vi "EdgeRegistration and ObjectTracking.vi"(8 "error in (no error)":errorcluster, 9 "Edge and object Parameters":T1={"Canny Edge Parameters"={"Sigma"=1.0, "HThresh"=0.7, "LThres"=0.2, "WindowSize"=9}, "Smoothing parameters"={"X Size"=3, "Y Size"=3, "% Tolerance"=40}, "Dilation iteration"=1, "Object recognition parameters"={"Objects"=0, "Threshold"=128, "Reject Border"=FALSE, "Fill Holes"=FALSE, "Min Object Size"=FALSE, "Min Size"=3, "Max Object Size"=FALSE, "Max Size"=100, "Show Search Area"=FALSE, "Show Center"=TRUE, "Show Bounding Box"=TRUE}} {"Object recognition parameters"."Objects" items=["Bright Objects", "Dark Objects"]; "Object recognition parameters"."Threshold" min=1 max=999999999 step=1; "Object recognition parameters"."Max Size" min=1 max=999999999 step=1; "Object recognition parameters"."Min Size" min=1 max=999999999 step=1; "Canny Edge Parameters"."LThres" min=0 max=1 format="%.2f"; "Canny Edge Parameters"."HThresh" min=0 max=1 format="%.2f"; "Canny Edge Parameters"."Sigma" min=0 max=1 format="%.2f"}, 10 "Roy":T2, 11 "Rob":T2) -> (0 "error out":errorcluster, 1 "Max value":dbl, 2 "y translation":dbl, 3 "x translation":dbl, 4 "object center y":sgl, 5 "object center X":sgl)   [LabVIEW 2012]
uses:
  <vilib>/vision/Image Controls.llb/IMAQ Image.ctl
  Edge and object parameters.ctl
  <vilib>/vision/NI_Vision_Development_Module.lvlib
panel:
  out "Edge cc":T2(plugin-control)
  out "Edge Roy":T2(plugin-control)
  out "Edge Rob":T2(plugin-control)
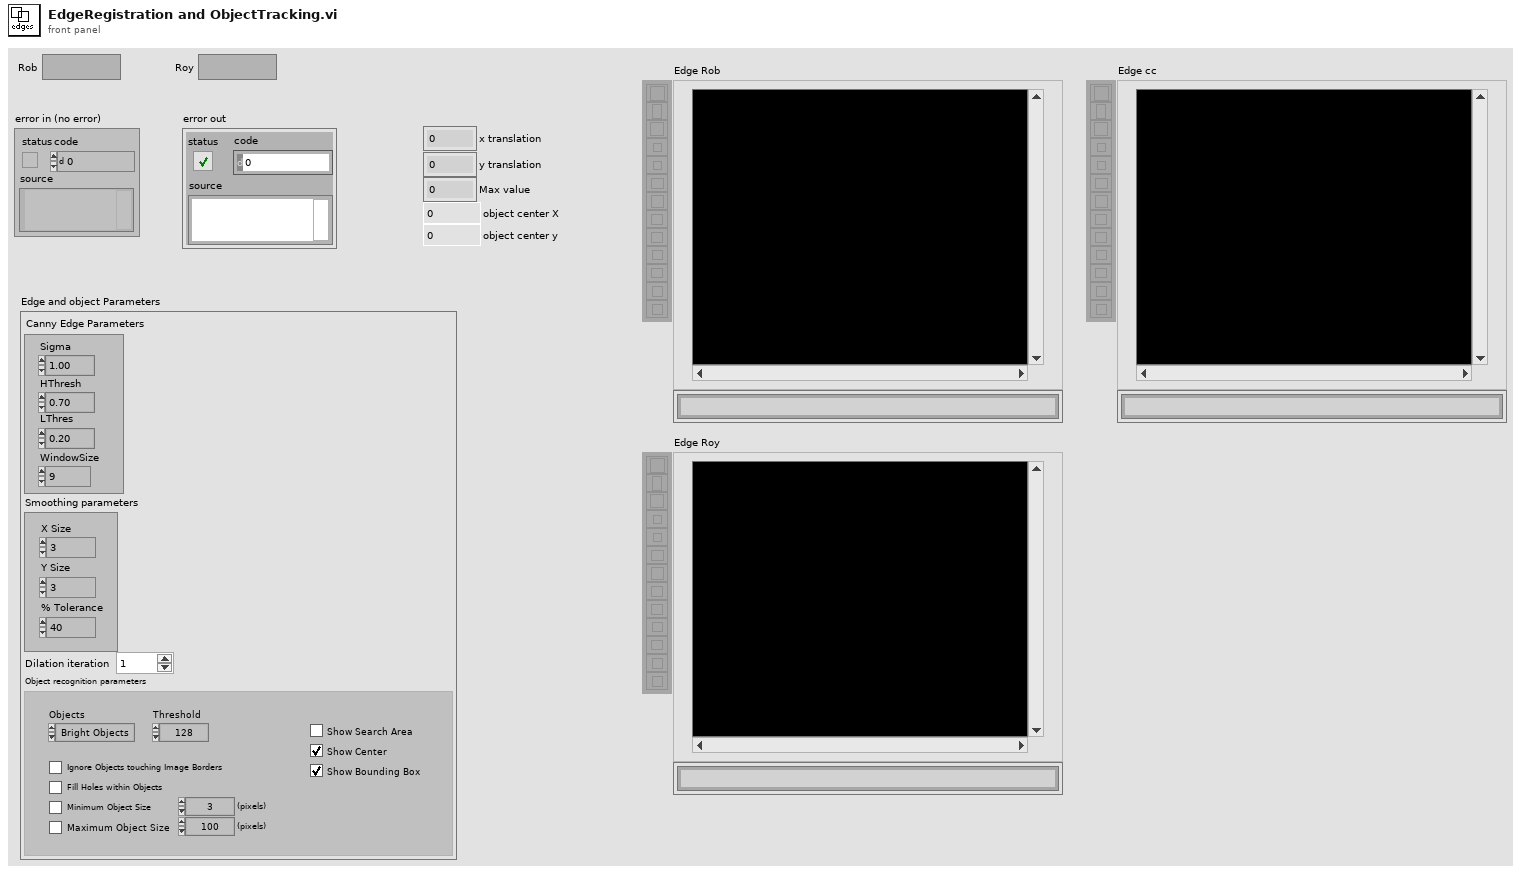
[diagram p1: front panel]
types:
  T1 = typedef "Edge and object parameters.ctl" = cluster{"Canny Edge Parameters":cluster{"Sigma":sgl, "HThresh":sgl, "LThres":sgl, "WindowSize":i32}, "Smoothing parameters":cluster{"X Size":i32, "Y Size":i32, "% Tolerance":i32}, "Dilation iteration":i32, "Object recognition parameters":cluster{"Objects":u16, "Threshold":i32, "Reject Border":bool, "Fill Holes":bool, "Min Object Size":bool, "Min Size":i32, "Max Object Size":bool, "Max Size":i32, "Show Search Area":bool, "Show Center":bool, "Show Bounding Box":bool}}
  T2 = typedef "IMAQ Image.ctl" = refnum<image>
  T3 = enum32{"AutoM", "Close", "Dilate", "Erode", "Gradient", "Gradient in", "Gradient out", "HitMiss", "Open", "PClose", "POpen", "Thick", "Thin"}
  T4 = cluster{"Sigma":sgl, "HThresh":sgl, "LThres":sgl, "WindowSize":i32}
  T5 = cluster{"X Size":i32, "Y Size":i32, "% Tolerance":i32}
  T6 = cluster{"Objects":u16, "Threshold":i32, "Reject Border":bool, "Fill Holes":bool, "Min Object Size":bool, "Min Size":i32, "Max Object Size":bool, "Max Size":i32, "Show Search Area":bool, "Show Center":bool, "Show Bounding Box":bool}
  T7 = cluster{"Object Center":cluster{"X":sgl, "Y":sgl}, "Bounding Box":cluster{"X Left":i32, "Y Top":i32, "X Right":i32, "Y Bottom":i32}, "Area":sgl, "Orientation":sgl, "Aspect Ratio":sgl, "Nb Holes":i32}[]
  T8 = cluster{"Object Center":cluster{"X":sgl, "Y":sgl}, "Bounding Box":cluster{"X Left":i32, "Y Top":i32, "X Right":i32, "Y Bottom":i32}, "Area":sgl, "Orientation":sgl, "Aspect Ratio":sgl, "Nb Holes":i32}
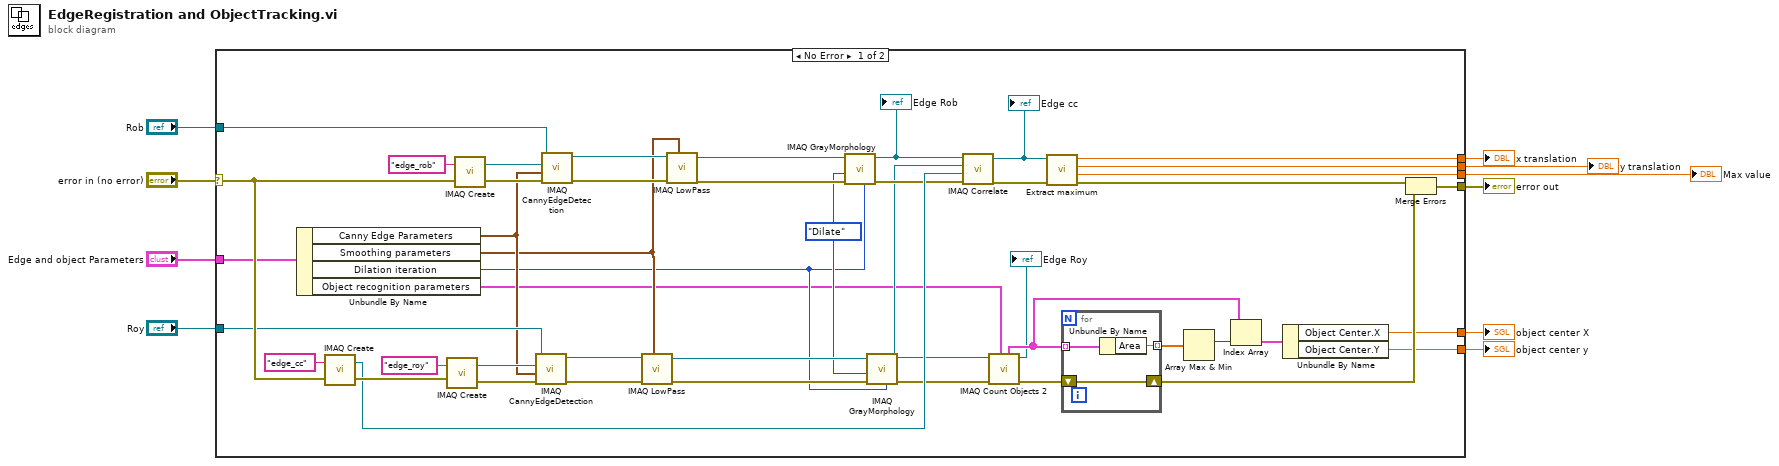
[diagram p0: block diagram]
diagram:
  n1 = case shown="No Error" "error in (no error)" {
    selector: "error in (no error)" -> [w46 w60]
    tunnel: "Rob" -> [w51 _]
    tunnel: "Roy" -> [w40 _]
    tunnel: [w31 _] -> w5
    tunnel: [w30 _] -> w4
    tunnel: [w29 _] -> w3
    tunnel: [w21 w60] -> w2
    tunnel: [w20 _] -> w7
    tunnel: [w19 _] -> w6
    tunnel: "Edge and object Parameters" -> [w18 _]
    frame No Error {
      w37 = T3."Dilate" ("Operation")
      n2 = Unbundle By Name(w18) -> ("Canny Edge Parameters"=w17:T4, "Smoothing parameters"=w16:T5, "Dilation iteration"=w15:i32, "Object recognition parameters"=w14:T6)
      n3 = call "IMAQ Create"("Image Name"="edge_cc", "error in (no error)"=w46) -> ("New Image"=w36:T2, "error out"=w45:errorcluster)  [unwired: 3 in]
      n4 = call "IMAQ Create"("Image Name"="edge_roy", "error in (no error)"=w45) -> ("New Image"=w41:T2, "error out"=w44:errorcluster)  [unwired: 3 in]
      n5 = call "IMAQ Create"("Image Name"="edge_rob", "error in (no error)"=w46) -> ("New Image"=w53:T2, "error out"=w52:errorcluster)  [unwired: 3 in]
      n6 = call "IMAQ CannyEdgeDetection"("Image Src"=w40, "Image Dst"=w41, "Filter Parameters"=w17, "error in (no error)"=w44) -> ("Image Dst Out"=w39:T2, "error out"=w43:errorcluster)  [unwired: 4 in]
      n7 = call "IMAQ CannyEdgeDetection"("Image Src"=w51, "Image Dst"=w53, "Filter Parameters"=w17, "error in (no error)"=w52) -> ("Image Dst Out"=w50:T2, "error out"=w49:errorcluster)  [unwired: 4 in]
      n8 = call "IMAQ LowPass"("Image Src"=w39, "Size & Tolerance"=w16, "error in (no error)"=w43) -> ("Image Dst Out"=w38:T2, "error out"=w42:errorcluster)  [unwired: 4 in]
      n9 = call "IMAQ LowPass"("Image Src"=w50, "Size & Tolerance"=w16, "error in (no error)"=w49) -> ("Image Dst Out"=w54:T2, "error out"=w48:errorcluster)  [unwired: 4 in]
      n10 = call "IMAQ GrayMorphology"("Number of iterations (1)"=w15, "error in (no error)"=w48, "Operation"=w37, "Image Src"=w54) -> ("error out"=w35:errorcluster, "Image Dst Out"=w13:T2)  [unwired: 6 in]
      "Edge Rob" <- w13
      n11 = call "IMAQ GrayMorphology"("Number of iterations (1)"=w15, "error in (no error)"=w42, "Operation"=w37, "Image Src"=w38) -> ("error out"=w32:errorcluster, "Image Dst Out"=w33:T2)  [unwired: 6 in]
      n12 = call "IMAQ Correlate"("Image Src"=w13, "Image Template"=w33, "Image Dst"=w36, "error in (no error)"=w35) -> ("Image Dst Out"=w12:T2, "error out"=w34:errorcluster)  [unwired: 3 in]
      "Edge cc" <- w12
      n13 = call "IMAQ Count Objects 2"("Settings"=w14, "error in (no error)"=w32, "Image"=w33) -> ("error out"=w28:errorcluster, "Image Out"=→"Edge Roy":T2, "Objects"=w25:T7)  [unwired: 4 in, 2 out]
      n14 = call "Extract maximum.vi"("error in (no error)"=w34, "Image in"=w12) -> ("error out"=w23:errorcluster, "Max value"=w29:dbl, "y translation"=w30:dbl, "x translation"=w31:dbl)  [unwired: 6 in]
      n15 = for {
        tunnel: w25 -> [w59] mode=indexing
        shift-right: [w57] -> w22
        shift-left: w28 -> [w57]
        tunnel: [w58] -> w27 mode=indexing
        n16 = Unbundle By Name(w59) -> ("Area"=w58:sgl)
      }
      n17 = Array Max & Min(array=w27) -> (max index (indices)=w26:i32)  [unwired: 3 out]
      n18 = Index Array(array=w25, index=w26) -> (element=w24:T8)
      n19 = Unbundle By Name(w24) -> ("Object Center.X"=w20:sgl, "Object Center.Y"=w19:sgl)
      n20 = Merge Errors(w23, w22) -> (w21:errorcluster)
    }
    frame Error {
    }
  }
  "x translation" <- w5
  "y translation" <- w4
  "Max value" <- w3
  "object center X" <- w7
  "object center y" <- w6
  "error out" <- w2
